vi "SetField_popup.vi"(4 "Field (T)":string="0", 5 "Rate (T/min)":string="0.3", 6 "error in (no error)":errorcluster, 7 "Input Line command":string) -> (0 "Output Line command":string, 2 "Cancel":bool, 3 "error out":errorcluster={"status"=TRUE, "code"=1, "source"="Scan From String (arg 1) in SetField.vi->main.vi"})   [LabVIEW 2020]
panel:
  in  "platform":u16(ring) items=["Mac", "PC"]
  in  "Cancel button":bool
  in  "OK Button":bool
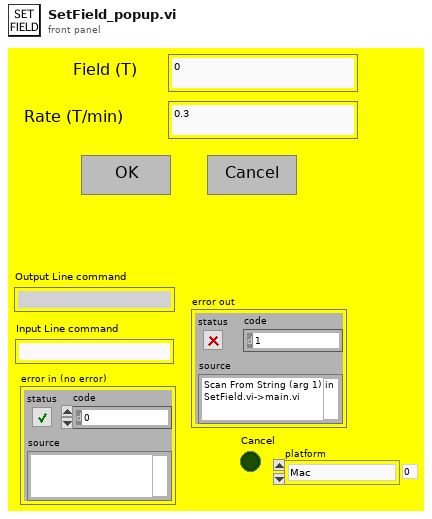
[diagram p1: front panel]
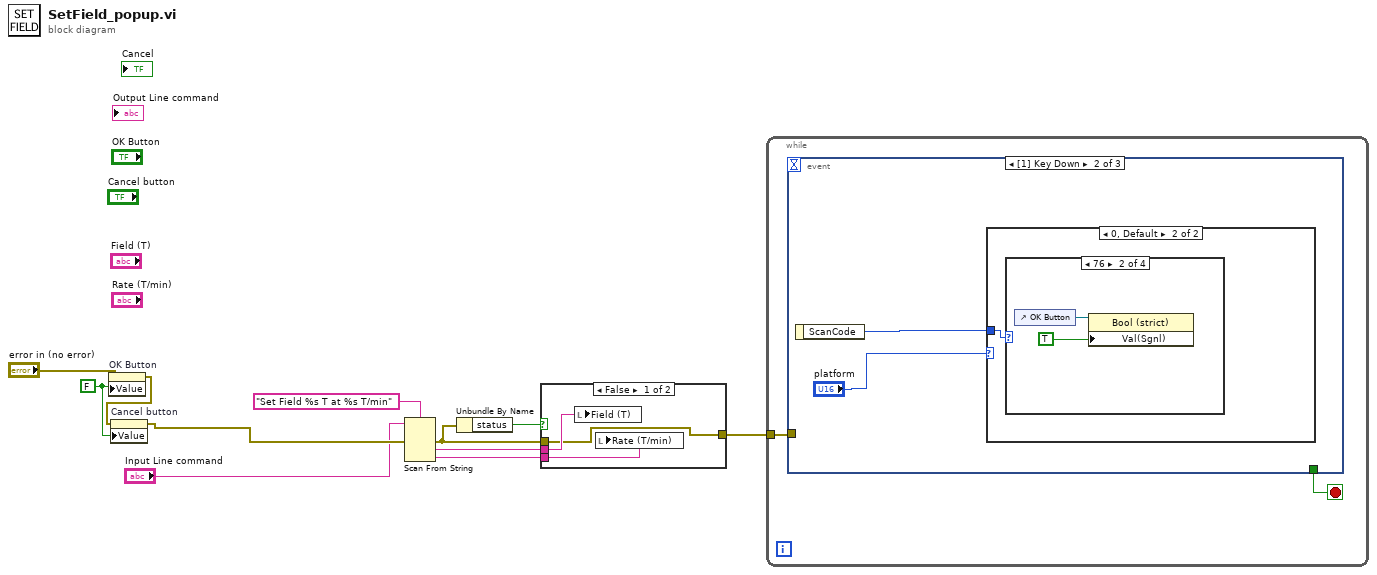
[diagram p0: block diagram]
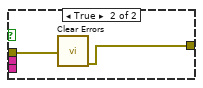
[diagram p2: hidden frame]
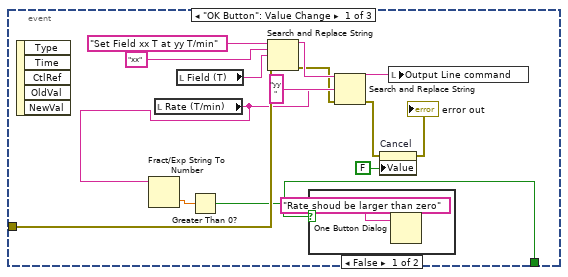
[diagram p3: hidden frame]
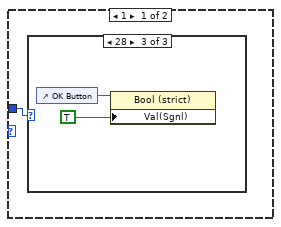
[diagram p5: hidden frame]
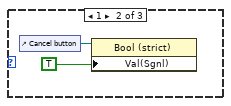
[diagram p7: hidden frame]
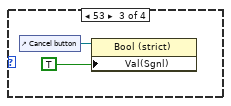
[diagram p9: hidden frame]
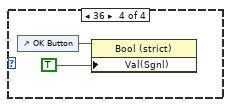
[diagram p10: hidden frame]
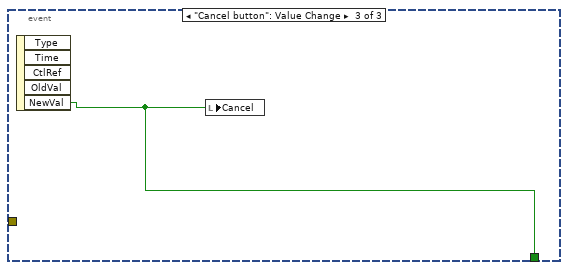
[diagram p11: hidden frame]
diagram:
  w11 = FALSE ("OK Button")
  n1 = property on="OK Button" class="Bool (strict)"(error in="error in (no error)", "Value"=w11) -> (error out=w10:errorcluster)  [unwired: 1 in, 1 out]
  n2 = property on="Cancel button" class="Bool (strict)"(error in=w10, "Value"=w11) -> (error out=w9:errorcluster)  [unwired: 1 in, 1 out]
  n3 = Scan From String(format string="Set Field %s T at %s T/min", input string="Input Line command", error in=w9) -> (error out=w3:errorcluster, output 1=w6:string, output 2=w5:string)  [unwired: 3 in, 2 out]
  n4 = Unbundle By Name(w3) -> ("status"=w4:bool)
  n5 = case shown="False" w4 {
    tunnel: w6 -> [w14 _]
    tunnel: w5 -> [w13 _]
    tunnel: w3 -> [w12 w16]
    tunnel: [w12 w15] -> w2
    frame False {
      n6 = local write "Field (T)"(w14) -> ()
      n7 = local write "Rate (T/min)"(w13) -> ()
    }
    frame True {
      n8 = call <vilib>:"Clear Errors.vi"("error in (no error)"=w16) -> ("error out"=w15:errorcluster)  [unwired: 5 in, 1 out]
    }
  }
  n9 = while {
    tunnel: w2 -> [w17]
    stop <- w18 stop-if-true
    n10 = event shown="[1] Key Down" {
      selector: _ -> [_ _ _]
      dyn-events: _ -> [_ _ _]
      timeout: _ -> [_ _ _]
      tunnel: [w19 _ w48] -> w18
      tunnel: w17 -> [w28 _ _]
      event "OK Button": Value Change {
        n11 = event-data() -> ()  [unwired: 1 in, 5 out]
        n12 = local read "Rate (T/min)"() -> (w21:string)
        n13 = Fract/Exp String To Number(string=w21) -> (number=w20:dbl)  [unwired: 3 in, 1 out]
        n14 = local read "Field (T)"() -> (w26:string)
        n15 = Greater Than 0?(x=w20) -> (x > 0?=w19:bool)
        n16 = Search and Replace String(input string="Set Field xx T at yy T/min", search string="xx", replace string=w26, error in=w28) -> (result string=w30:string, error out=w27:errorcluster)  [unwired: 4 in, 2 out]
        n17 = case shown="False" w19 {
          frame False {
            n18 = One Button Dialog(message="Rate shoud be larger than zero") -> ()  [unwired: 1 in, 1 out]
          }
          frame True {
          }
        }
        n19 = Search and Replace String(input string=w30, search string="yy", replace string=w21, error in=w27) -> (result string=w23:string, error out=w25:errorcluster)  [unwired: 4 in, 2 out]
        n20 = property on="Cancel" class="Bool (strict)"(error in=w25, "Value"=FALSE ("Cancel")) -> (error out=→"error out":errorcluster)  [unwired: 1 in, 1 out]
        n21 = local write "Output Line command"(w23) -> ()
      }
      event Key Down {
        n22 = event-data() -> ("ScanCode"=w35:i16)  [unwired: 1 in]
        n23 = case shown="0, Default" "platform" {
          tunnel: w35 -> [w36 w41]
          frame 1 {
            n24 = case shown="28" w36 {
              frame Default {
              }
              frame 1 {
                n25 = control-ref of="Cancel button"() -> (w37:refnum<vi>)
                n26 = property on="Property Node" class="Bool (strict)"(reference=w37, "Val(Sgnl)"=TRUE) -> ()  [unwired: 1 in, 2 out]
              }
              frame 28 {
                n27 = control-ref of="OK Button"() -> (w39:refnum<vi>)
                n28 = property on="Property Node" class="Bool (strict)"(reference=w39, "Val(Sgnl)"=TRUE) -> ()  [unwired: 1 in, 2 out]
              }
            }
          }
          frame 0, Default {
            n29 = case shown="76" w41 {
              frame Default {
              }
              frame 76 {
                n30 = control-ref of="OK Button"() -> (w42:refnum<vi>)
                n31 = property on="Property Node" class="Bool (strict)"(reference=w42, "Val(Sgnl)"=TRUE) -> ()  [unwired: 1 in, 2 out]
              }
              frame 53 {
                n32 = control-ref of="Cancel button"() -> (w44:refnum<vi>)
                n33 = property on="Property Node" class="Bool (strict)"(reference=w44, "Val(Sgnl)"=TRUE) -> ()  [unwired: 1 in, 2 out]
              }
              frame 36 {
                n34 = control-ref of="OK Button"() -> (w46:refnum<vi>)
                n35 = property on="Property Node" class="Bool (strict)"(reference=w46, "Val(Sgnl)"=TRUE) -> ()  [unwired: 1 in, 2 out]
              }
            }
          }
        }
      }
      event "Cancel button": Value Change {
        n36 = event-data() -> ("NewVal"=w48:bool)  [unwired: 1 in, 4 out]
        n37 = local write "Cancel"(w48) -> ()
      }
    }
  }
